vi "DoesPathMatchOldFileName.vi"(10 "Old File Name":string, 11 "File Path":path) -> (2 "Match Found":bool, 3 "Parent Directory":path)   [LabVIEW 2024]
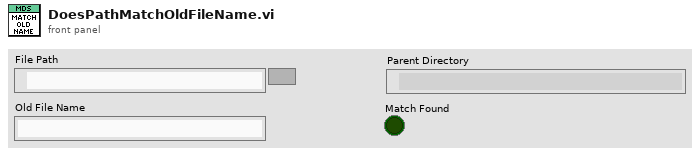
[diagram p1: front panel]
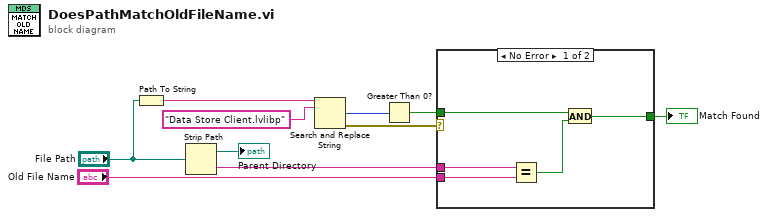
[diagram p0: block diagram]
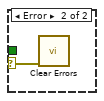
[diagram p2: hidden frame]
diagram:
  n1 = Path To String(path="File Path") -> (string=w9:string)
  n2 = Strip Path(path="File Path") -> (stripped path=→"Parent Directory":path, name=w3:string)
  n3 = Search and Replace String(input string=w9, search string="Data Store Client.lvlibp") -> (number of replacements=w6:i32, error out=w7:errorcluster)  [unwired: 6 in, 2 out]
  n4 = Greater Than 0?(x=w6) -> (x > 0?=w5:bool)
  n5 = case shown="No Error" w7 {
    selector: w7 -> [_ w16]
    tunnel: w5 -> [w13 _]
    tunnel: "Old File Name" -> [w15 _]
    tunnel: w3 -> [w14 _]
    tunnel: [w11 _] -> w2
    frame No Error {
      n6 = Equal?(x=w14, y=w15) -> (x = y?=w12:bool)
      n7 = And(x=w13, y=w12) -> (x .and. y?=w11:bool)
    }
    frame Error {
      n8 = call <vilib>:"Clear Errors.vi"("error in (no error)"=w16) -> ()  [unwired: 5 in, 2 out]
    }
  }
  "Match Found" <- w2
